vi "DigitsToNum(U16).vi"(8 "error in (no error)":errorcluster caption="错误输入（无错误）", 10 "基数 (10)":u16=10, 11 "位数数组":u16[](array[numeric])) -> (0 "error out":errorcluster caption="错误输出", 3 "数值":u16)   [LabVIEW 2012]
doc: "Converts a single I32 into an array of digits, in order of increasing significance. If the input number is negative, the most significant digit (last element of the array) is also negative. All other digits are always non-negative. By default, the output digits are the digits used to represent the number in base 10, though the base can be changed. For example, the binary representation can be obtained by wiring the value 2 to the Base input. Note that Base is coerced to a minimum value of 2.\n\nAs long as no coersion is required, the original number can be recreated as\nN = Digits[0] * Base^0 + Digits[1] * Base^1 + Digits[2] * Base^2 + ... + Digits[n] * Base^n\n\nFreeware from Moore Good Ideas, www.mooregoodideas.com. Do not remove this line."
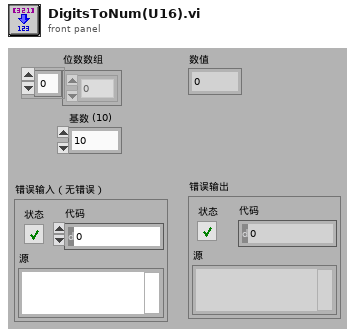
[diagram p1: front panel]
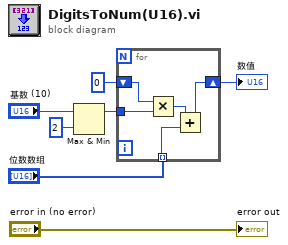
[diagram p0: block diagram]
diagram:
  n1 = Max & Min(x="基数 (10)", y=u16 2) -> (max(x,y)=w4:u16)  [unwired: 1 out]
  n2 = for {
    tunnel: "位数数组" -> [w9] mode=indexing
    tunnel: w4 -> [w12]
    shift-right: [w8] -> w2
    shift-left: u16 0 ("y") -> [w11]
    n3 = Multiply(x=w11, y=w12) -> (x*y=w10:u16)
    n4 = Add(x=w10, y=w9) -> (x+y=w8:u16)
  }
  "数值" <- w2
  "error out" <- "error in (no error)"
